vi "DAC Run.vi"(8 "error in":errorcluster, 11 "DAC Pump Inv in":refnum<class "DAC Pump Inv.lvclass">) -> (0 "error out":errorcluster, 3 "DAC Pump Inv out":refnum<class "DAC Pump Inv.lvclass">)   [LabVIEW 2019, in "DAC.lvlib" / "DAC Pump Inv.lvclass"]
uses:
  DAC Pump Inv.lvclass
  DAC.lvclass
  Results/Results Method.ctl
  Results/Results.lvlib
  <vilib>/DAQmx/write.llb/DAQmx Write (Analog DBL 1Chan 1Samp).vi
  Results/Water Tunnel Results/Water Tunnel Results.lvclass
  C:/Users/wg/Documents/LV_Projects/test-stand/App/DAC/DAC.lvclass
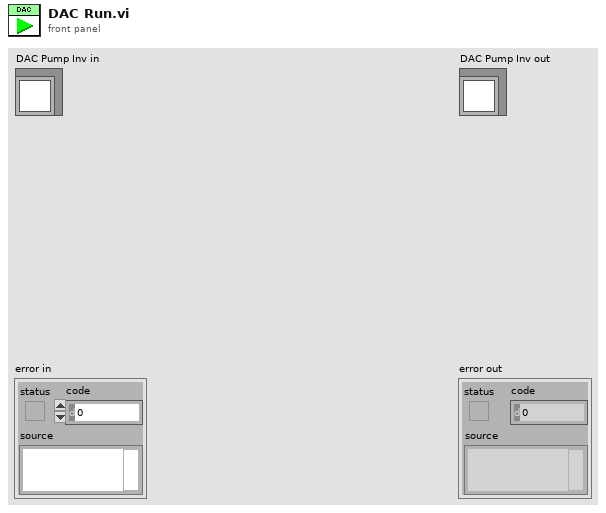
[diagram p1: front panel]
types:
  T1 = typedef "Results.lvlib/Results Method.ctl" = enum16{"Get", "Set"}
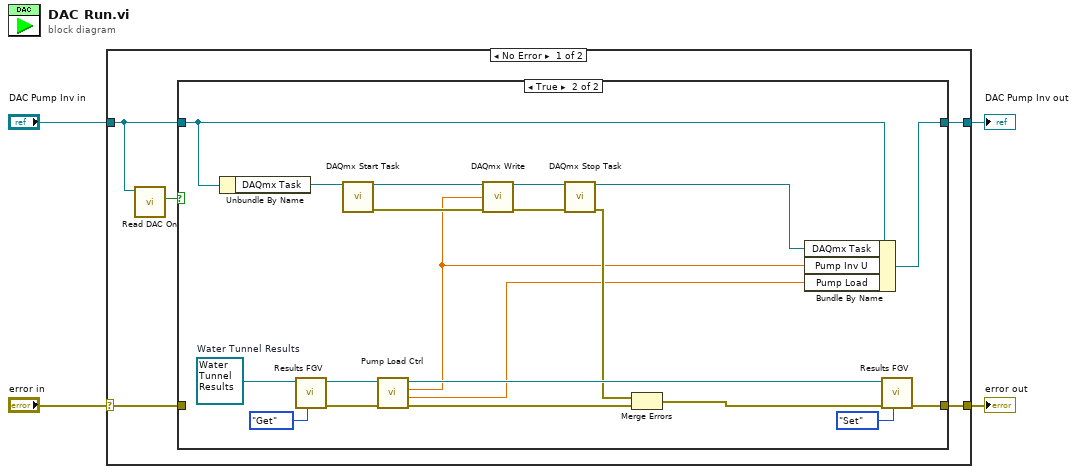
[diagram p0: block diagram]
diagram:
  n1 = case shown="No Error" "error in" {
    selector: "error in" -> [w7 w33]
    tunnel: [w6 w33] -> w2
    tunnel: [w8 w32] -> w1
    tunnel: "DAC Pump Inv in" -> [w5 w32]
    frame No Error {
      n2 = call "Read DAC On.vi"("DAC in"=w5) -> ("DAC On"=w9:bool)  [unwired: 8 in, 2 out]
      n3 = case shown="True" w9 {
        tunnel: w5 -> [w11 w27]
        tunnel: [w11 w22] -> w8
        tunnel: w7 -> [w10 _]
        tunnel: [w10 w21] -> w6
        frame False {
        }
        frame True {
          w20 = refnum<class "Water Tunnel Results.lvclass"> refnum  # Water Tunnel Results
          n4 = Unbundle By Name(w27) -> ("DAQmx Task"=w31:refnum<k21>)
          n5 = call-dynamic "Results FGV.vi"("Method"=Results_Method."Get", "Water Tunnel Results in"=w20) -> ("error out"=w17:errorcluster, "Water Tunnel  Results out"=w19:refnum<class "Water Tunnel Results.lvclass">)  [unwired: 8 in]
          n6 = call <vilib>:"DAQmx Start Task.vi"("task/channels in"=w31) -> ("task out"=w30:refnum<k21>, "error out"=w29:errorcluster)  [unwired: 13 in]
          n7 = call "Pump Load Ctrl.vi"("error in"=w17, "Water Tunnel Results in"=w19) -> ("error out"=w15:errorcluster, "Pump Load"=w12:dbl, "Pump Inv U"=w13:dbl, "Water Tunnel Results out"=w18:refnum<class "Water Tunnel Results.lvclass">)  [unwired: 6 in]
          n8 = call-poly <vilib>:"DAQmx Write.vi"("task/channels in"=w30, "data"=w13, "error in"=w29) -> ("task out"=w23:refnum<k21>, "error out"=w28:errorcluster)  [unwired: 10 in, 1 out]
          n9 = call <vilib>:"DAQmx Stop Task.vi"("task/channels in"=w23, "error in"=w28) -> ("task out"=w24:refnum<k21>, "error out"=w16:errorcluster)  [unwired: 12 in]
          n10 = Merge Errors(w16, w15) -> (w14:errorcluster)
          n11 = Bundle By Name(cluster=w27, "DAQmx Task"=w24, "Pump Inv U"=w13, "Pump Load"=w12) -> (w22:refnum<class "DAC Pump Inv.lvclass">)
          n12 = call-dynamic "Results FGV.vi"("Method"=Results_Method."Set", "error in"=w14, "Water Tunnel Results in"=w18) -> ("error out"=w21:errorcluster)  [unwired: 7 in, 1 out]
        }
      }
    }
    frame Error {
    }
  }
  "error out" <- w2
  "DAC Pump Inv out" <- w1
